vi "TestStepsGui.Steps.FormatStatus.vi"(10 "Status":T1) -> (2 "Status str":string)   [LabVIEW 2016]
uses:
  Sequence/Sequence.Step.Status.ctl
  tools/Translator/Translator.Global.vi
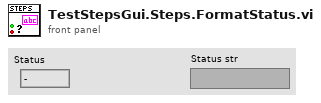
[diagram p1: front panel]
types:
  T1 = typedef "Sequence.Step.Status.ctl" = enum16{"-", "Pending", "Running", "Skipped", "Passed", "Failed", "Done", "Error", "Aborted", "Stopped"}
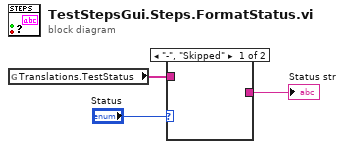
[diagram p0: block diagram]
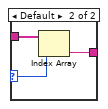
[diagram p2: hidden frame]
diagram:
  n1 = global read "Translator.Global.vi" "Translations.TestStatus"() -> (w1:string[])
  n2 = case shown="\"-\", \"Skipped\"" "Status" {
    selector: "Status" -> [_ w5]
    tunnel: [_ w4] -> w3
    tunnel: w1 -> [_ w6]
    frame "-", "Skipped" {
    }
    frame Default {
      n3 = Index Array(array=w6, index=w5) -> (element=w4:string)
    }
  }
  "Status str" <- w3
